vi "RangeI2C-array-single.vi"() -> ()   [LabVIEW 2014]
panel:
  in  "Array of Addresses":i32[](array[numeric])=[200, 224]
  out "Array of Ranges":dbl[](array[numeric])
  in  "Remote Port":u16=502
  in  "Remote IP Address":string="192.168.124.53"
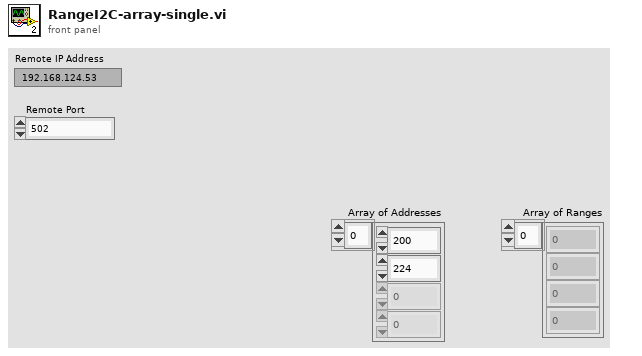
[diagram p1: front panel]
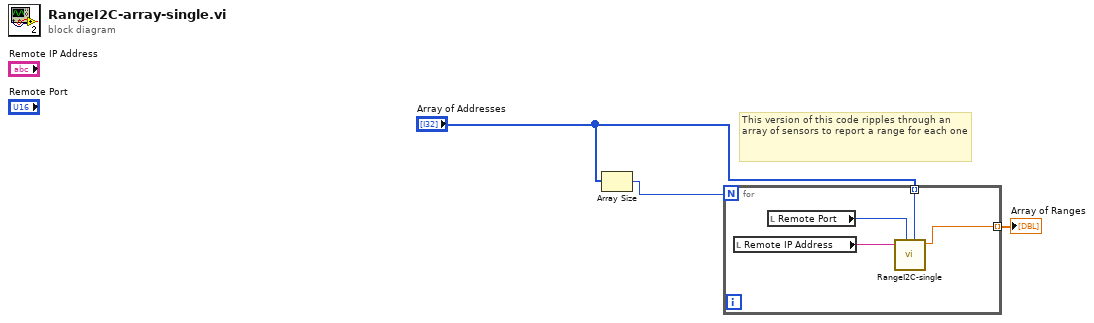
[diagram p0: block diagram]
diagram:
  # "This version of this code ripples through an array of sensors to report a range for each one"
  n1 = Array Size(array="Array of Addresses") -> (size(s)=w3:i32)
  n2 = for {
    N: w3 -> [_]
    tunnel: "Array of Addresses" -> [w5] mode=indexing
    tunnel: [w4] -> w1 mode=indexing
    n3 = local read "Remote IP Address"() -> (w7:string)
    n4 = local read "Remote Port"() -> (w6:u16)
    n5 = call "RangeI2C-single.vi"("Remote IP Address"=w7, "Remote Port"=w6, "CURRENT 8-bit address (dec.)"=w5) -> ("Range (cm)"=w4:dbl)  [unwired: 6 in, 1 out]
  }
  "Array of Ranges" <- w1
